vi "Smart text logger.vi"(8 "Message":string, 9 "Logs in":string[](array[string])) -> (1 "Logs out":string[](array[string]))   [LabVIEW 2021, in "MatS Libs.lvlib"]
doc: "Shifts old logs and puts new \"<date> <time>_<message>\" on top (start of array). If the message repeates more than twice, only the date and time are changd to the current one in the top"
uses:
  <userlib>/MatS Libs/MatS Libs.lvlib
panel:
  out "Repeats twice?":bool
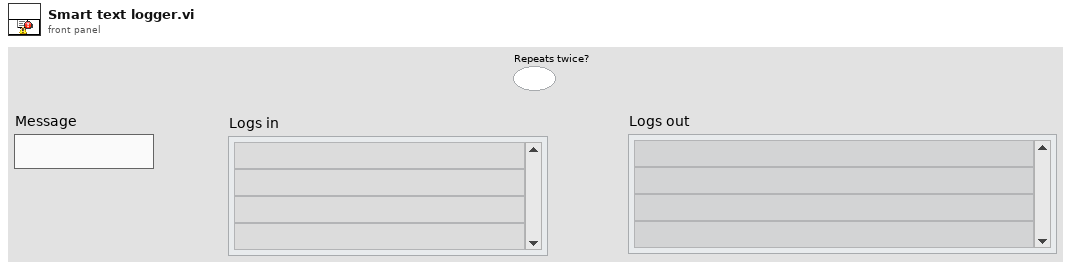
[diagram p1: front panel]
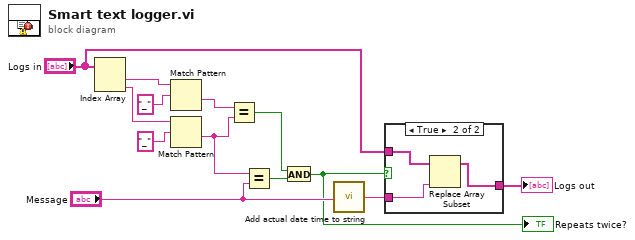
[diagram p0: block diagram]
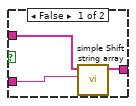
[diagram p2: hidden frame]
diagram:
  n1 = Index Array(array="Logs in") -> (element #1=w13:string, element #2=w8:string)  [unwired: 2 in]
  n2 = Match Pattern(string=w13, regular expression="_") -> (after substring=w7:string)  [unwired: 1 in, 3 out]
  n3 = Match Pattern(string=w8, regular expression="_") -> (after substring=w6:string)  [unwired: 1 in, 3 out]
  n4 = Equal?(x=w7, y=w6) -> (x = y?=w3:bool)
  n5 = Equal?(x=w6, y="Message") -> (x = y?=w4:bool)
  n6 = And(x=w3, y=w4) -> (x .and. y?=w5:bool)
  "Repeats twice?" <- w5
  n7 = call <userlib>:"Add actual date time to string.vi"("String in"="Message") -> ("String out"=w2:string)  [unwired: 4 in]
  n8 = case shown="True" w5 {
    tunnel: [w16 w17] -> w1
    tunnel: "Logs in" -> [w15 w19]
    tunnel: w2 -> [w14 w18]
    frame False {
      n9 = call <userlib>:"simple Shift string array.vi"("Element in"=w14, "Array in"=w15) -> ("Array out"=w16:string[])  [unwired: 8 in, 1 out]
    }
    frame True {
      n10 = Replace Array Subset(array=w19, new element=w18) -> (w17:string[])  [unwired: 1 in]
    }
  }
  "Logs out" <- w1
